vi "CFTS-Init State.vi"(0 "Experimenter":string, 1 "Root folder":path, 5 "Num":i32, 7 "Right":string, 9 "Left":string) -> (4 "State (out)":T1, 15 "error out":errorcluster)   [LabVIEW 2020]
doc: "Initializes ABI experiment state based on the specified experiment ID."
uses:
  CFTS-Experiment State.ctl
  CFTS-Globals.vi
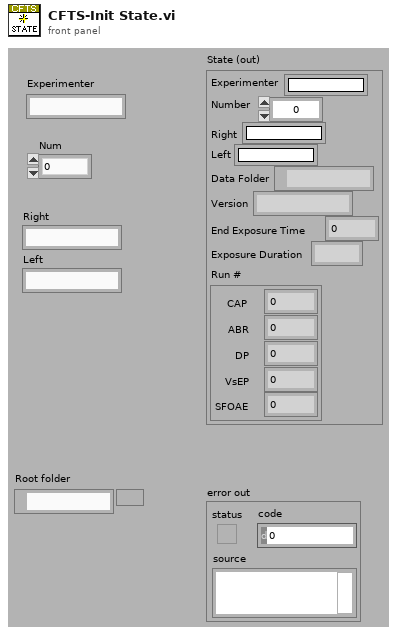
[diagram p1: front panel]
types:
  T1 = typedef "CFTS-Experiment State.ctl" = cluster{"Experimenter":string, "Number":u32, "Right":string, "Left":string, "Data Folder":path, "Version":string, "End Exposure Time":dbl, "Exposure Duration":string, "Run #":cluster{"CAP":i32, "ABR":i32, "DP":i32, "VsEP":i32, "SFOAE":i32}}
  T2 = cluster{"CAP":i16, "ABR":i16, "DP":i16, "VsEP":i16, "MeasSeq 3":i16}
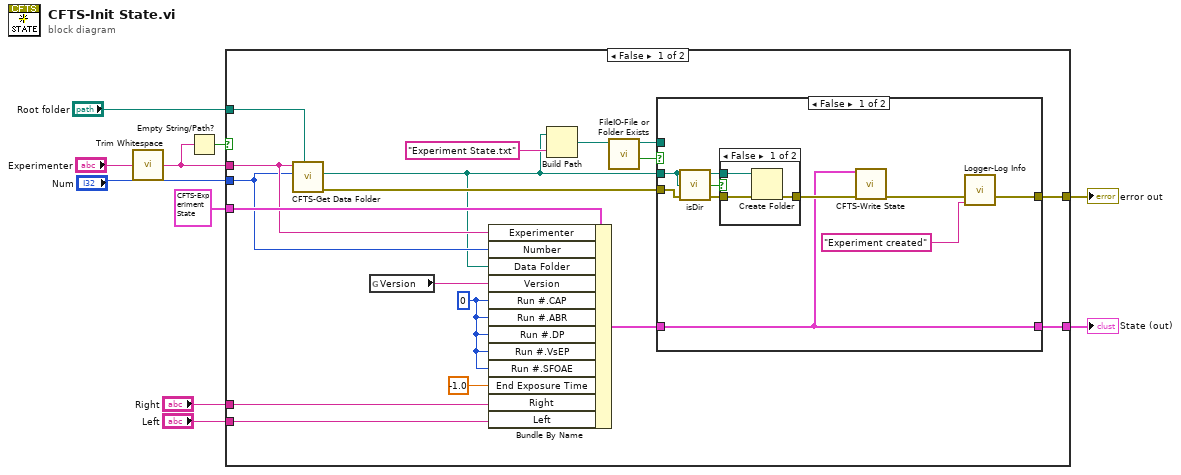
[diagram p0: block diagram]
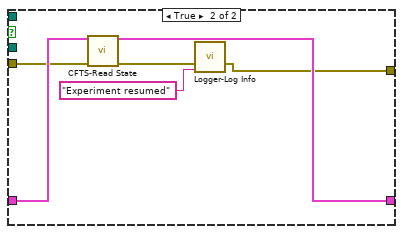
[diagram p3: hidden frame]
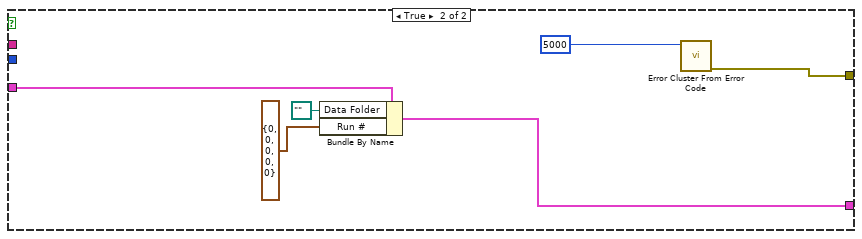
[diagram p4: hidden frame]
diagram:
  n1 = call <vilib>:"Trim Whitespace.vi"("string"="Experimenter") -> ("trimmed string"=w8:string)  [unwired: 1 in]
  n2 = Empty String/Path?(string/path=w8) -> (empty?=w9:bool)
  n3 = case shown="False" w9 {
    tunnel: T1 {"Experimenter"="", "Number"=0, "Right"="", "Left"="", "Data Folder"=path "", "Version"="", "End Exposure Time"=0.0, "Exposure Duration"="", "Run #"={"CAP"=0, "ABR"=0, "DP"=0, "VsEP"=0, "SFOAE"=0}} ("State") -> [w28 w52]
    tunnel: [w24 w49] -> w7
    tunnel: w8 -> [w25 _]
    tunnel: "Num" -> [w16 _]
    tunnel: [w23 w51] -> w10
    tunnel: "Root folder" -> [w20 _]
    tunnel: "Left" -> [w18 _]
    tunnel: "Right" -> [w17 _]
    frame False {
      w21 = 0 ("Next run #")
      n4 = call "CFTS-Get Data Folder.vi"("Root folder"=w20, "Number"=w16, "Experimenter"=w25) -> ("error out"=w22:errorcluster, "Data folder"=w14:path)  [unwired: 7 in]
      n5 = global read "CFTS-Globals.vi" "Version"() -> (w19:string)
      n6 = Bundle By Name(cluster=w28, "Experimenter"=w25, "Number"=w16, "Data Folder"=w14, "Version"=w19, "Run #.CAP"=w21, "Run #.ABR"=w21, "Run #.DP"=w21, "Run #.VsEP"=w21, "Run #.SFOAE"=w21, "End Exposure Time"=-1.0, "Right"=w17, "Left"=w18) -> (w27:T1)
      n7 = Build Path(base path=w14, name or relative path="Experiment State.txt" ("subkey")) -> (appended path=w13:path)
      n8 = call "FileIO-File or Folder Exists.vi"("path"=w13) -> ("Exists?"=w12:bool, "dup path"=w11:path)  [unwired: 7 in, 2 out]
      n9 = case shown="False" w12 {
        tunnel: w14 -> [w34 _]
        tunnel: [w31 w42] -> w24
        tunnel: w27 -> [w32 w46]
        tunnel: [w32 w44] -> w23
        tunnel: w22 -> [w35 w45]
        tunnel: w11 -> [_ _]
        frame False {
          n10 = call "isDir.vi"("path"=w34) -> ("is Dir?"=w33:bool)
          n11 = case shown="False" w33 {
            tunnel: [w39 w40] -> w36
            tunnel: w35 -> [w38 w40]
            tunnel: w34 -> [w37 _]
            frame False {
              n12 = Create Folder(path (use dialog)=w37, error in=w38) -> (error out=w39:errorcluster)  [unwired: 1 in, 2 out]
            }
            frame True {
            }
          }
          n13 = call "CFTS-Write State.vi"("State"=w32, "error in (no error)"=w36) -> ("error out"=w29:errorcluster)  [unwired: 12 in, 1 out]
          n14 = call "Logger-Log Info.vi"("error in (no error)"=w29, "Message"="Experiment created" ("message")) -> ("error out"=w31:errorcluster)  [unwired: 13 in]
        }
        frame True {
          n15 = call "CFTS-Read State.vi"("State In"=w46, "error in (no error)"=w45) -> ("State Out"=w44:T1, "error out"=w43:errorcluster)  [unwired: 12 in]
          n16 = call "Logger-Log Info.vi"("error in (no error)"=w43, "Message"="Experiment resumed" ("message")) -> ("error out"=w42:errorcluster)  [unwired: 13 in]
        }
      }
    }
    frame True {
      n17 = Bundle By Name(cluster=w52, "Data Folder"=path "", "Run #"=T2 {"CAP"=0, "ABR"=0, "DP"=0, "VsEP"=0, "MeasSeq 3"=0}) -> (w51:T1)
      n18 = call <vilib>:"Error Cluster From Error Code.vi"("error code (0)"=5000) -> ("error out"=w49:errorcluster)  [unwired: 8 in]
    }
  }
  "State (out)" <- w10
  "error out" <- w7
